vi "TDMSFormatGroupProperties.vi"(0 "mL given":dbl, 1 "Go Trial Probability":dbl, 3 "RingText.Text":string, 5 "NRewards":i32, 7 "Session Performance":dbl, 9 "Trial Counter":i32, 11 "Training Duration (ms)":u32, 12 "Punishment Period (s)":i32, 13 "Airpuff (ms)":u32=400, 14 "Response Window (ms)":u32) -> (4 "Property Values":string[](array[string]), 6 "Property names":string[](array[string]))   [LabVIEW 2013]
panel:
  out "Label.Text":string
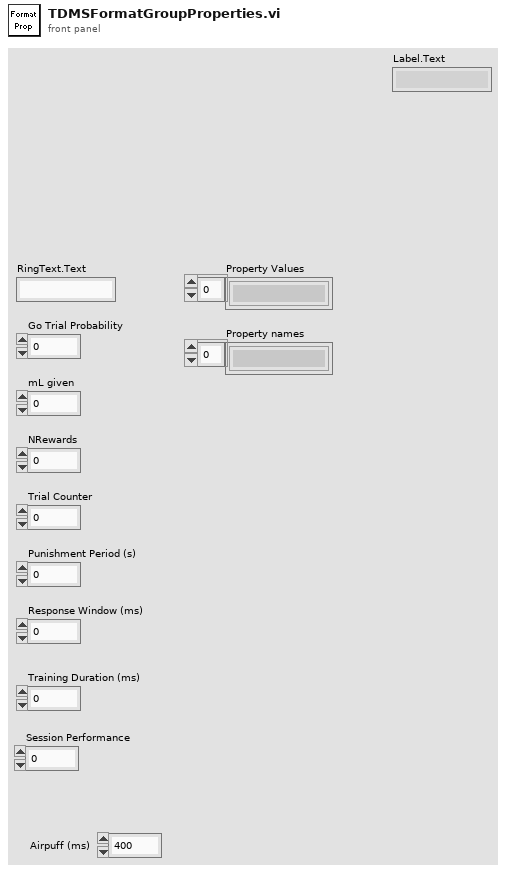
[diagram p1: front panel]
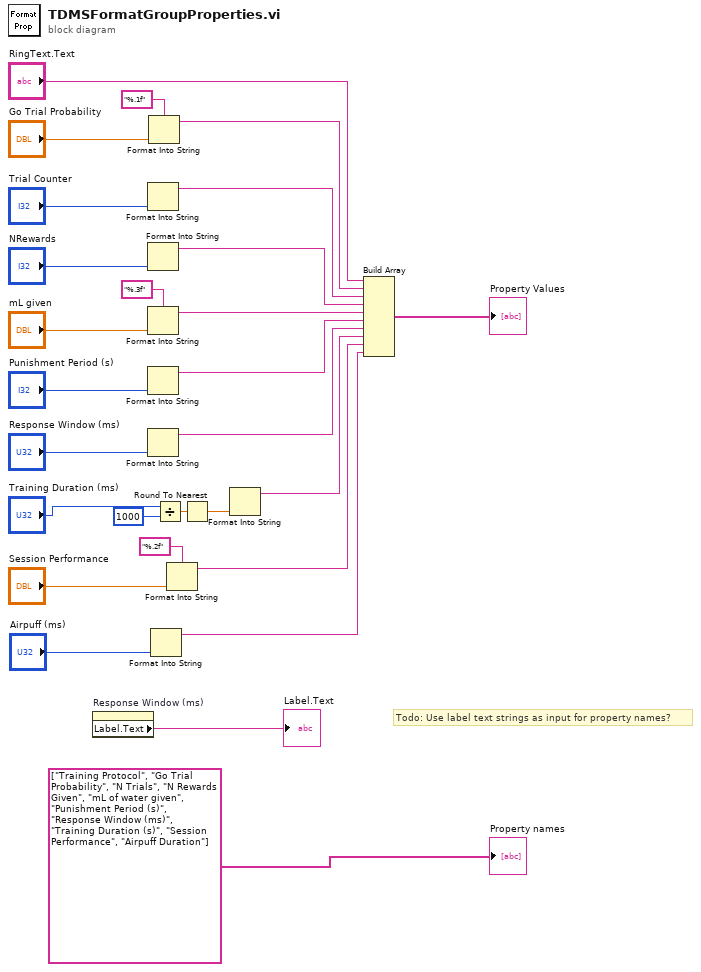
[diagram p0: block diagram]
diagram:
  # "Todo: Use label text strings as input for property names?"
  n1 = property on="Response Window (ms)" class="DigNum (strict)"() -> ("Label.Text"=→"Label.Text":string)  [unwired: 2 in, 2 out]
  n2 = Format Into String("Trial Counter") -> (resulting string=w24:string)  [unwired: 3 in, 1 out]
  n3 = Format Into String("NRewards") -> (resulting string=w22:string)  [unwired: 3 in, 1 out]
  n4 = Format Into String(format string="%.3f", "mL given") -> (resulting string=w21:string)  [unwired: 2 in, 1 out]
  n5 = Format Into String("Punishment Period (s)") -> (resulting string=w27:string)  [unwired: 3 in, 1 out]
  n6 = Format Into String("Response Window (ms)") -> (resulting string=w28:string)  [unwired: 3 in, 1 out]
  n7 = Format Into String(format string="%.1f", "Go Trial Probability") -> (resulting string=w17:string)  [unwired: 2 in, 1 out]
  n8 = Format Into String("Airpuff (ms)") -> (resulting string=w1:string)  [unwired: 3 in, 1 out]
  n9 = Divide(x="Training Duration (ms)", y=u32 1000) -> (x/y=w8:dbl)
  n10 = Format Into String(format string="%.2f", "Session Performance") -> (resulting string=w3:string)  [unwired: 2 in, 1 out]
  n11 = Round To Nearest(number=w8) -> (nearest integer value=w7:dbl)
  n12 = Format Into String(w7) -> (resulting string=w6:string)  [unwired: 3 in, 1 out]
  n13 = Build Array("RingText.Text", w17, w24, w22, w21, w27, w28, w6, w3, w1) -> (→"Property Values":string[])
  "Property names" <- string[] ["Training Protocol", "Go Trial Probability", "N Trials", "N Rewards Given", "mL of water given", "Punishment Period (s)", "Response Window (ms)", "Training Duration (s)", "Session Performance", "Airpuff Duration"] ("property names")
